vi "Get time.vi"(8 "error in (no error)":errorcluster) -> (0 "error out":errorcluster, 3 "time out":timestamp)   [LabVIEW 2020]
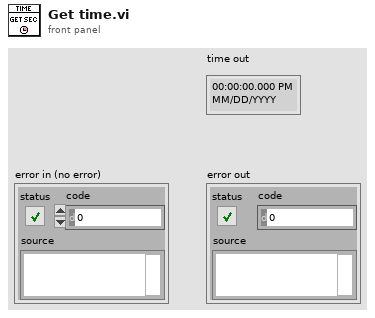
[diagram p1: front panel]
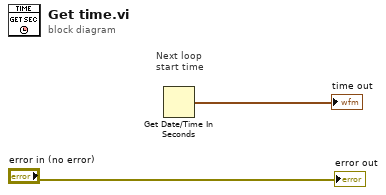
[diagram p0: block diagram]
diagram:
  # "Next loop start time"
  n1 = Get Date/Time In Seconds() -> (seconds since 1Jan1904=→"time out":timestamp)
  "error out" <- "error in (no error)"
